vi "Get Error out from Terminals Info.vi"(11 "terminals info":T1) -> (2 "error out terms indexes":i32[](array[numeric]), 3 "error out wires":refnum<vi>[](array[refnum]))   [LabVIEW 2014]
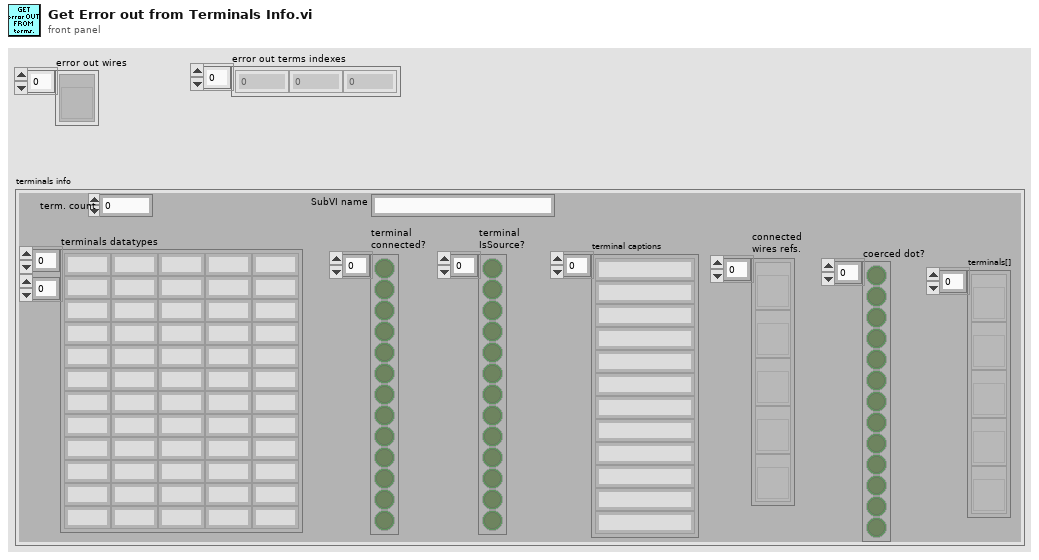
[diagram p1: front panel]
types:
  T1 = cluster{"terminals datatypes":string[][], "terminal\nconnected?":bool[], "terminal captions":string[], "term. count":i32, "terminal\nIsSource?":bool[], "SubVI name":string, "connected\nwires refs.":refnum<vi>[], "coerced dot?":bool[], "terminals[]":refnum<vi>[]}
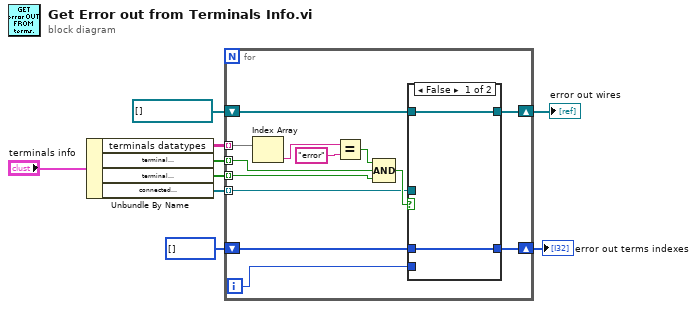
[diagram p0: block diagram]
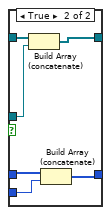
[diagram p2: hidden frame]
diagram:
  n1 = Unbundle By Name("terminals info") -> ("terminals datatypes"=w8:string[][], "terminal\nIsSource?"=w7:bool[], "terminal\nconnected?"=w3:bool[], "connected\nwires refs."=w5:refnum<vi>[])
  n2 = for {
    tunnel: w8 -> [w22] mode=indexing
    tunnel: w7 -> [w18] mode=indexing
    shift-right: [w14] -> w4
    shift-left: refnum<vi>[] [] ("connected\nwires refs.") -> [w16]
    tunnel: w5 -> [w15] mode=indexing
    tunnel: w3 -> [w13] mode=indexing
    shift-right: [w11] -> w1
    shift-left: i32[] [] -> [w10]
    i -> [w12]
    n3 = Index Array(array=w22) -> (element=w21:string)  [unwired: 1 in]
    n4 = Equal?(x=w21, y="error") -> (x = y?=w19:bool)
    n5 = Compound Arithmetic op=AND(w19, w18, w13) -> (w17:bool)
    n6 = case shown="False" w17 {
      tunnel: [w24 w29] -> w14
      tunnel: w16 -> [w24 w30]
      tunnel: w15 -> [_ w28]
      tunnel: [w23 w25] -> w11
      tunnel: w12 -> [_ w27]
      tunnel: w10 -> [w23 w26]
      frame False {
      }
      frame True {
        n7 = Build Array (concatenate)(w30, w28) -> (w29:refnum<vi>[])
        n8 = Build Array (concatenate)(w26, w27) -> (w25:i32[])
      }
    }
  }
  "error out wires" <- w4
  "error out terms indexes" <- w1
